vi "MotorPos2WL.vi"(1 "Mono2 Motor Position":dbl) -> (0 "Mono2 Center Wavelength (nm)":dbl)   [LabVIEW 2019]
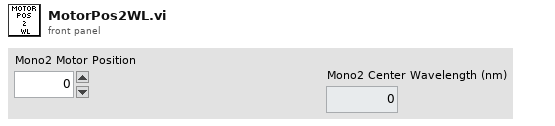
[diagram p1: front panel]
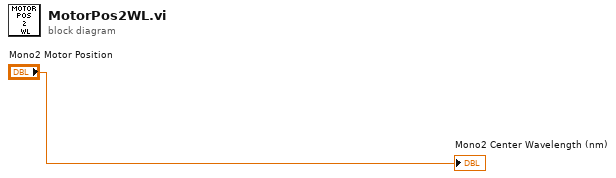
[diagram p0: block diagram]
diagram:
  "Mono2 Center Wavelength (nm)" <- "Mono2 Motor Position"
